vi "MM9.RemoveSystemNames.vi"(0 "i ref in":refnum<vi>, 3 "ms timeout (10000)":i32=10000, 5 "error in (no error)":errorcluster) -> (14 "i ref out":refnum<vi>, 17 "timed out":bool, 19 "error out":errorcluster)   [LabVIEW 2014, in "MM9.lvlib"]
doc: "This vi updates the list of used objects stored in the MassMeas attribute."
uses:
  MM9.lvlib
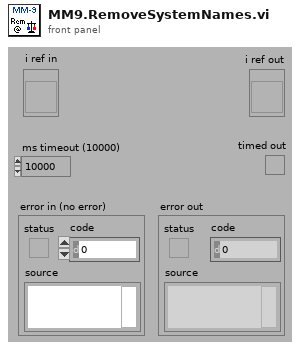
[diagram p1: front panel]
types:
  T1 = typedef "MM9.lvlib/MM9.i attribute.ctl" = cluster{"UsedObjs":string[], "ActScanStep":i32[], "AbortRequest":bool, "StopRequest":bool, "# cycles":i32, "Connected":bool, "MMStatus":T2, "# data":i32, "DIMServices":cluster{"MM6StatusString":string, "MM6StatusID":i32, "discArchiver":string, "discArchiverID":i32, "eventBuilder":string, "eventBuilderID":i32, "GUIIDString":string, "GUIIDStringID":i32}, "dataFile":string, "PGRunning":T3, "ConfigData":T4, "ExtraDataSets":T19}
  T2 = typedef "MM9.lvlib/MM9.status.ctl" = enum16{"loaded", "load_error", "config", "config_error", "init", "init_error", "data_reset", "data_reset_error", "running", "start_error", "run_error", "abort_requested", "aborted", "stop_requested", "stopped", "stop_error", "Connected", "NOTConnected"}
  T3 = typedef "PPG_ABC.lvlib/PPG_ABC.PG_Running.ctl" = i32
  T4 = typedef "LEBITDefs9.lvlib/LEBITDefs.ConfigData.ctl" = cluster{"GenConfig":T5, "Configs":T7[]}
  T5 = typedef "LEBITDefs9.lvlib/LEBITDefs.GenConfig.ctl" = cluster{"Mode":i32, "Logs":T6[]}
  T6 = typedef "LEBITDefs9.lvlib/LEBITDefs.Log.ctl" = cluster{"Name":string, "FctName":string, "Special":string}
  T7 = typedef "LEBITDefs9.lvlib/LEBITDefs.OneConfig.ctl" = cluster{"MCA":T8, "Timing":T9, "Scans":T12[], "FreqDevs":T13[], "CleanDev":T14, "NrCycles":i32, "Specials":T16[], "Delays":T17[], "DAC":T18}
  T8 = typedef "LEBITDefs9.lvlib/LEBITDefs.MCA.ctl" = cluster{"Name":string, "Address":string, "NrChannels":i32, "Gate":i32, "NrPipse":i32, "AcqDelay":i32}
  T9 = typedef "LEBITDefs9.lvlib/LEBITDefs.Timing.ctl" = cluster{"TimeTables":cluster{"TimeTable":T10}[], "Memories":T11[], "ScanX":string, "ScanY":string}
  T10 = typedef "LEBITDefs9.lvlib/LEBITDefs.Timetable.ctl" = dbl[]
  T11 = typedef "LEBITDefs9.lvlib/LEBITDefs.Memory.ctl" = cluster{"Device":string, "ExtTrig":bool, "TT2Use":i32, "PatternTable":string[]}
  T12 = typedef "LEBITDefs9.lvlib/LEBITDefs.ScanDev.ctl" = cluster{"Name":string, "FctName":string, "Values":dbl[], "NrScanVals":i32, "Special":string}
  T13 = typedef "LEBITDefs9.lvlib/LEBITDefs.FreqDev.ctl" = cluster{"Name":string, "Amp":dbl, "CenterFreq":dbl, "Time":dbl}
  T14 = typedef "LEBITDefs9.lvlib/LEBITDefs.CleanDev.ctl" = cluster{"Name":string, "CleanData":T15[]}
  T15 = typedef "LEBITDefs9.lvlib/LEBITDefs.CleanDataType.ctl" = cluster{"Amp":dbl, "Center":dbl, "Plus":dbl, "Minus":dbl, "Time":dbl}
  T16 = typedef "LEBITDefs9.lvlib/LEBITDefs.Special.ctl" = cluster{"Name":string, "FctName":string, "VerySpecial":string, "Data":dbl}
  T17 = typedef "LEBITDefs9.lvlib/LEBITDefs.Delay.ctl" = cluster{"Name":string, "Delay":dbl}
  T18 = typedef "LEBITDefs9.lvlib/LEBITDefs.DAC.ctl" = cluster{"Name":string, "Step1":i32, "Step2":i32}
  T19 = typedef "LEBITDefs9.lvlib/LEBITDefs.ExtraData.ctl" = cluster{"Ions":cluster{"ExcitIonMass":string, "ExcitIonCharge":i32, "CleanIons":cluster{"CleanIonMass":string, "CleanIonCharge":i32}[]}, "TimingDescription":cluster{"TimeTableDescription":cluster{"Times":string[]}[], "PatternTableDescription":cluster{"Pattern":string[]}[]}, "ScanUnits":string[]}[]
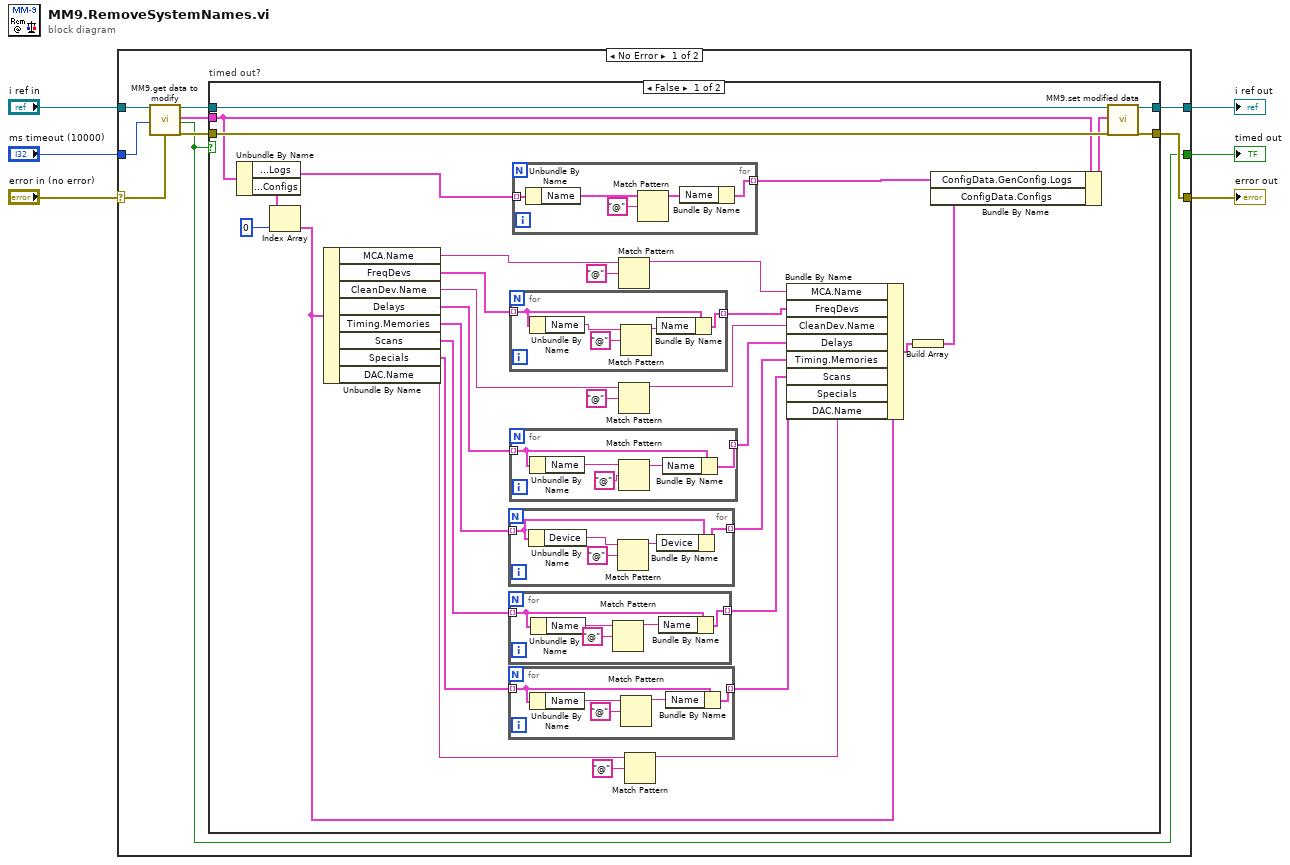
[diagram p0: block diagram]
diagram:
  n1 = case shown="No Error" "error in (no error)" {
    selector: "error in (no error)" -> [w7 w80]
    tunnel: "i ref in" -> [w15 w81]
    tunnel: [w14 w80] -> w5
    tunnel: [w13 w81] -> w4
    tunnel: "ms timeout (10000)" -> [w9 _]
    tunnel: [w8 _] -> w2
    frame No Error {
      n2 = call "MM9.get data to modify.vi"("i ref in"=w15, "ms timeout (10000)"=w9, "error in (no error)"=w7) -> ("i ref out"=w12:refnum<vi>, "i attribute"=w10:T1, "timed out"=w8:bool, "error out"=w11:errorcluster)  [unwired: 13 in]
      n3 = case "timed out?" shown="False" w8 {
        tunnel: [w47 w78] -> w14
        tunnel: [w46 w79] -> w13
        tunnel: w12 -> [w45 w79]
        tunnel: w11 -> [w44 w78]
        tunnel: w10 -> [w27 _]
        frame False {
          n4 = Unbundle By Name(w27) -> ("ConfigData.GenConfig.Logs"=w37:T6[], "ConfigData.Configs"=w38:T7[])
          n5 = Index Array(array=w38, index=0) -> (element=w35:T7)
          n6 = Unbundle By Name(w35) -> ("MCA.Name"=w24:string, "FreqDevs"=w39:T13[], "CleanDev.Name"=w21:string, "Delays"=w43:T17[], "Timing.Memories"=w42:T11[], "Scans"=w41:T12[], "Specials"=w40:T16[], "DAC.Name"=w17:string)
          n7 = for {
            tunnel: w42 -> [w72] mode=indexing
            tunnel: [w71] -> w31 mode=indexing
            n8 = Unbundle By Name(w72) -> ("Device"=w68:string)
            n9 = Match Pattern(string=w68, regular expression="@") -> (before substring=w69:string)  [unwired: 1 in, 3 out]
            n10 = Bundle By Name(cluster=w72, "Device"=w69) -> (w71:T11)
          }
          n11 = for {
            tunnel: w41 -> [w67] mode=indexing
            tunnel: [w66] -> w30 mode=indexing
            n12 = Unbundle By Name(w67) -> ("Name"=w64:string)
            n13 = Match Pattern(string=w64, regular expression="@") -> (before substring=w63:string)  [unwired: 1 in, 3 out]
            n14 = Bundle By Name(cluster=w67, "Name"=w63) -> (w66:T12)
          }
          n15 = for {
            tunnel: w40 -> [w62] mode=indexing
            tunnel: [w61] -> w29 mode=indexing
            n16 = Unbundle By Name(w62) -> ("Name"=w59:string)
            n17 = Match Pattern(string=w59, regular expression="@") -> (before substring=w58:string)  [unwired: 1 in, 3 out]
            n18 = Bundle By Name(cluster=w62, "Name"=w58) -> (w61:T16)
          }
          n19 = for {
            tunnel: w39 -> [w57] mode=indexing
            tunnel: [w56] -> w34 mode=indexing
            n20 = Unbundle By Name(w57) -> ("Name"=w54:string)
            n21 = Match Pattern(string=w54, regular expression="@") -> (before substring=w53:string)  [unwired: 1 in, 3 out]
            n22 = Bundle By Name(cluster=w57, "Name"=w53) -> (w56:T13)
          }
          n23 = for {
            tunnel: w43 -> [w77] mode=indexing
            tunnel: [w76] -> w32 mode=indexing
            n24 = Unbundle By Name(w77) -> ("Name"=w74:string)
            n25 = Match Pattern(string=w74, regular expression="@") -> (before substring=w73:string)  [unwired: 1 in, 3 out]
            n26 = Bundle By Name(cluster=w77, "Name"=w73) -> (w76:T17)
          }
          n27 = for {
            tunnel: w37 -> [w52] mode=indexing
            tunnel: [w51] -> w26 mode=indexing
            n28 = Unbundle By Name(w52) -> ("Name"=w48:string)
            n29 = Match Pattern(string=w48, regular expression="@") -> (before substring=w49:string)  [unwired: 1 in, 3 out]
            n30 = Bundle By Name(cluster=w52, "Name"=w49) -> (w51:T6)
          }
          n31 = Match Pattern(string=w24, regular expression="@") -> (before substring=w23:string)  [unwired: 1 in, 3 out]
          n32 = Match Pattern(string=w21, regular expression="@") -> (before substring=w20:string)  [unwired: 1 in, 3 out]
          n33 = Match Pattern(string=w17, regular expression="@") -> (before substring=w18:string)  [unwired: 1 in, 3 out]
          n34 = Bundle By Name(cluster=w35, "MCA.Name"=w23, "FreqDevs"=w34, "CleanDev.Name"=w20, "Delays"=w32, "Timing.Memories"=w31, "Scans"=w30, "Specials"=w29, "DAC.Name"=w18) -> (w33:T7)
          n35 = Build Array(w33) -> (w28:T7[])
          n36 = Bundle By Name(cluster=w27, "ConfigData.GenConfig.Logs"=w26, "ConfigData.Configs"=w28) -> (w36:T1)
          n37 = call "MM9.set modified data.vi"("i ref in"=w45, "i attribute"=w36, "error in (no error)"=w44) -> ("i ref out"=w46:refnum<vi>, "error out"=w47:errorcluster)  [unwired: 15 in]
        }
        frame True {
        }
      }
    }
    frame Error {
    }
  }
  "error out" <- w5
  "i ref out" <- w4
  "timed out" <- w2
